vi "GetDigitalInput.vi"(4 "error in (no error)":errorcluster, 6 "digital input configuration":u16(ring)=15 items=["Negative Limit Switch"=0, "Positive Limit Switch"=1, "Home Switch"=2, "Position Marker"=3, "Drive Enable"=4, "Quick Stop"=5, "General Purpose A"=15, "General Purpose B"=14, "General Purpose C"=13, "General Purpose D"=12, "General Purpose E"=11, "General Purpose F"=10, "General Purpose G"=9, "General Purpose H"=8], 7 "axis in":cluster{"keyHandle":u32, "nodeId":u16}={"keyHandle"=0, "nodeId"=1}) -> (0 "error out":errorcluster, 2 "active state":bool, 3 "axis out":cluster{"keyHandle":u32, "nodeId":u16}={"keyHandle"=0, "nodeId"=1})   [LabVIEW 2019, in "maxonEPOS.lvlib"]
doc: "<B>GetDigitalInput</B> reads one digital input state from the device."
uses:
  Examples/maxonEPOS.lvlib
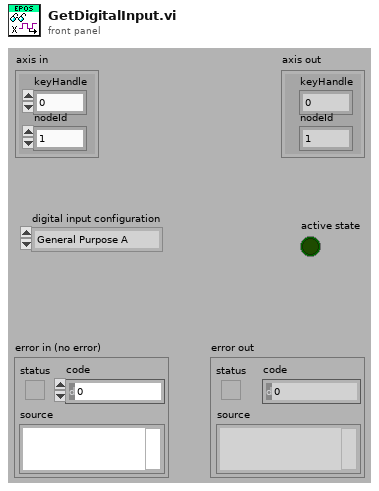
[diagram p1: front panel]
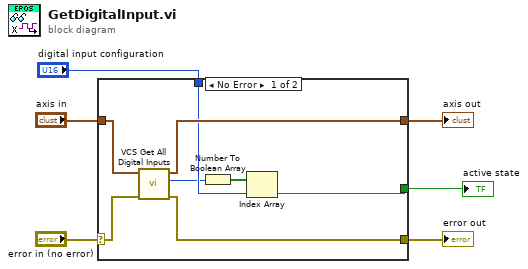
[diagram p0: block diagram]
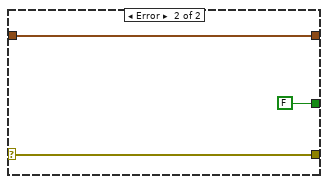
[diagram p2: hidden frame]
diagram:
  n1 = case shown="No Error" "error in (no error)" {
    selector: "error in (no error)" -> [w13 w17]
    tunnel: [w11 w17] -> w5
    tunnel: [w12 w16] -> w4
    tunnel: "axis in" -> [w14 w16]
    tunnel: "digital input configuration" -> [w10 _]
    tunnel: [w7 FALSE] -> w1
    frame No Error {
      n2 = call "VCS Get All Digital Inputs.vi"("error in (no error)"=w13, "axis in"=w14) -> ("error out"=w11:errorcluster, "digital inputs"=w8:u16, "axis out"=w12:cluster{"keyHandle":u32, "nodeId":u16})  [unwired: 7 in]
      n3 = Number To Boolean Array(number=w8) -> (Boolean array=w9:bool[])
      n4 = Index Array(array=w9, index=w10) -> (element=w7:bool)
    }
    frame Error {
    }
  }
  "error out" <- w5
  "axis out" <- w4
  "active state" <- w1
